vi "Auto 9.vi"(8 "Error In":errorcluster) -> (0 "Error Out":errorcluster)   [LabVIEW 2014]
uses:
  <vilib>/Rock Robotics/Network Tables/SD Read Boolean.vi
  <vilib>/Rock Robotics/Network Tables/SD Read Number.vi
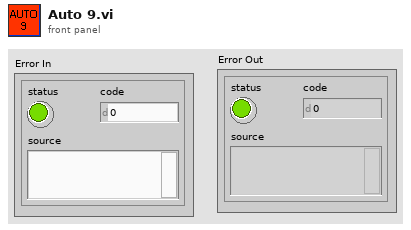
[diagram p1: front panel]
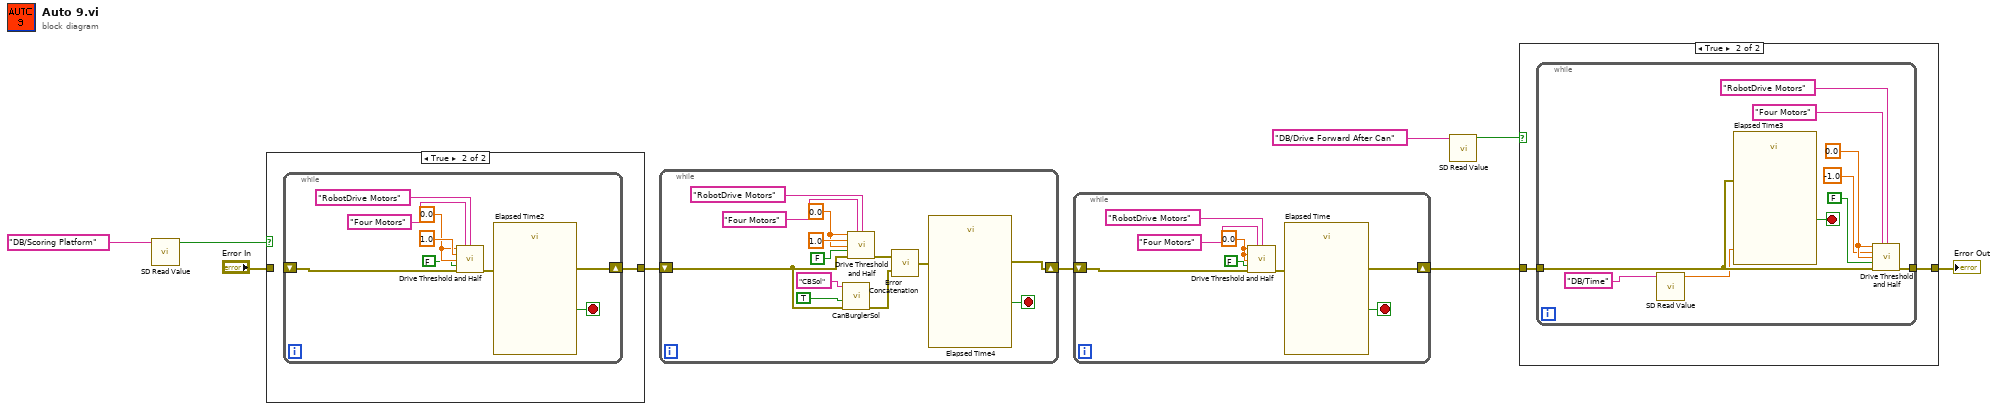
[diagram p0: block diagram]
diagram:
  n1 = call-poly <vilib>:"SD Read Value.vi"("Name"="DB/Scoring Platform") -> ("Boolean"=w3:bool)  [unwired: 8 in, 2 out]
  n2 = case shown="True" w3 {
    tunnel: "Error In" -> [w10 _]
    tunnel: [w10 w11] -> w1
    frame False {
    }
    frame True {
      n3 = while {
        shift-right: [w13] -> w11
        shift-left: _ -> [w14]
        stop <- w20 stop-if-true
        w18 = 0.0 ("Arm Value")
        n4 = call "Drive Threshold and Half.vi"("X In"=w18, "Drive refnum name"="Four Motors" ("refnum name"), "Send to DB Name"="RobotDrive Motors" ("Name"), "Y In"=1.0 ("X In"), "R In"=w18, "Speed Toggle"=FALSE ("Grabber Open/Close"), "Error In"=w14) -> ("Error Out"=w12:errorcluster)  [unwired: 8 in]
        n5 = call "Elapsed Time2"("error in (no error)"=w12) -> ("Time has Elapsed"=w20:bool, "error out"=w13:errorcluster)  [unwired: 11 in, 6 out]
      }
    }
  }
  n6 = while {
    shift-right: [w21] -> w2
    shift-left: w1 -> [w25]
    stop <- w31 stop-if-true
    w29 = 0.0 ("Arm Value")
    n7 = call "CanBurglerSol.vi"("Error In"=w25, "Grabber Open/Close"=TRUE, "refnum name"="CBSol") -> ("Error Out"=w23:errorcluster)  [unwired: 8 in]
    n8 = call "Drive Threshold and Half.vi"("X In"=w29, "Drive refnum name"="Four Motors" ("refnum name"), "Send to DB Name"="RobotDrive Motors" ("Name"), "Y In"=1.0 ("X In"), "R In"=w29, "Speed Toggle"=FALSE ("Grabber Open/Close"), "Error In"=w25) -> ("Error Out"=w24:errorcluster)  [unwired: 8 in]
    n9 = call "Error Concatenation.vi"("error in (no error) 2"=w23, "error in (no error)"=w24) -> ("error out"=w22:errorcluster)
    n10 = call "Elapsed Time4"("error in (no error)"=w22) -> ("Time has Elapsed"=w31:bool, "error out"=w21:errorcluster)  [unwired: 11 in, 6 out]
  }
  n11 = while {
    shift-right: [w36] -> w7
    shift-left: w2 -> [w37]
    stop <- w41 stop-if-true
    w34 = 0.0 ("Arm Value")
    n12 = call "Drive Threshold and Half.vi"("X In"=w34, "Drive refnum name"="Four Motors" ("refnum name"), "Send to DB Name"="RobotDrive Motors" ("Name"), "Y In"=w34, "R In"=w34, "Speed Toggle"=FALSE ("Grabber Open/Close"), "Error In"=w37) -> ("Error Out"=w35:errorcluster)  [unwired: 8 in]
    n13 = call "Elapsed Time"("error in (no error)"=w35) -> ("Time has Elapsed"=w41:bool, "error out"=w36:errorcluster)  [unwired: 11 in, 6 out]
  }
  n14 = call-poly <vilib>:"SD Read Value.vi"("Name"="DB/Drive Forward After Can") -> ("Boolean"=w5:bool)  [unwired: 8 in, 2 out]
  n15 = case shown="True" w5 {
    tunnel: w7 -> [w42 w44]
    tunnel: [w42 w43] -> w9
    frame False {
    }
    frame True {
      n16 = while {
        tunnel: [w51] -> w43
        tunnel: w44 -> [w48]
        stop <- w49 stop-if-true
        w50 = 0.0 ("Arm Value")
        n17 = call-poly <vilib>:"SD Read Value.vi"("Name"="DB/Time") -> ("Numeric"=w46:dbl)  [unwired: 8 in, 2 out]
        n18 = call "Elapsed Time3"("Time Target (s)"=w46, "error in (no error)"=w48) -> ("Time has Elapsed"=w49:bool)  [unwired: 10 in, 7 out]
        n19 = call "Drive Threshold and Half.vi"("X In"=w50, "Drive refnum name"="Four Motors" ("refnum name"), "Send to DB Name"="RobotDrive Motors" ("Name"), "Y In"=-1.0 ("X In"), "R In"=w50, "Speed Toggle"=FALSE ("Grabber Open/Close"), "Error In"=w48) -> ("Error Out"=w51:errorcluster)  [unwired: 8 in]
      }
    }
  }
  "Error Out" <- w9
